vi "Window-Restart window.vi"(8 "error in (no error)":errorcluster) -> (0 "error out":errorcluster, 1 "Cancelled (Left button pressed)":bool)   [LabVIEW 2017]
doc: "Use this template to create a dialog box with event handling."
uses:
  <vilib>/Utility/miscctls.llb/LVPointTypeDef.ctl
  Global Variables/General Globals.vi
panel:
  in  "Left Button":bool
  in  "Rigth Button":bool
  # "Confirm software restart"
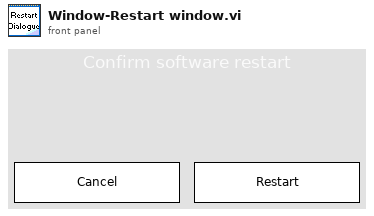
[diagram p1: front panel]
types:
  T1 = typedef "LVPointTypeDef.ctl" = cluster{"Horizontal":i16, "Vertical":i16}
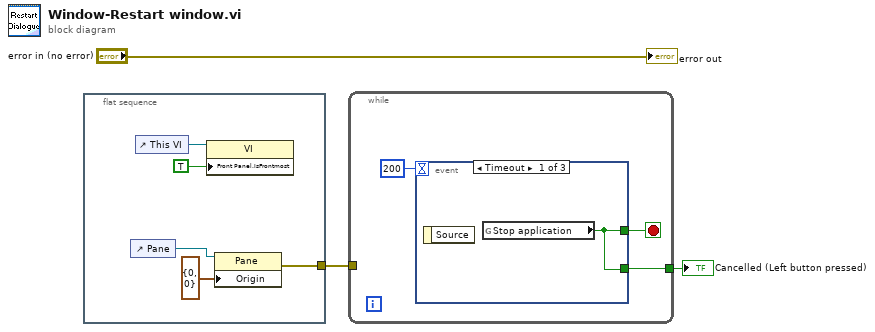
[diagram p0: block diagram]
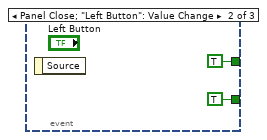
[diagram p2: hidden frame]
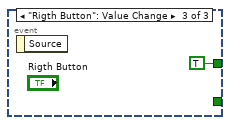
[diagram p3: hidden frame]
diagram:
  n1 = flat-sequence {
    tunnel: [w5] -> w3
    frame #0 {
      n2 = control-ref of="Pane"() -> (w4:refnum<vi>)
      n3 = control-ref of="This VI"() -> (w7:refnum<vi>)
      n4 = property on="Property Node" class="VI"(reference=w7, "Front Panel.IsFrontmost"=TRUE ("Front Panel Window:Is Frontmost")) -> ()  [unwired: 1 in, 2 out]
      n5 = property class="Pane"(reference=w4, "Origin"=T1 {"Horizontal"=0, "Vertical"=0}) -> (error out=w5:errorcluster)  [unwired: 1 in, 1 out]
    }
  }
  n6 = while {
    tunnel: w3 -> [_]
    tunnel: [w9] -> w2
    stop <- w11 stop-if-true
    n7 = event shown="[0] Timeout" {
      selector: _ -> [_ _ _]
      dyn-events: _ -> [_ _ _]
      timeout: 200 -> [_ _ _]
      tunnel: [w12 TRUE ("Stop?") TRUE ("Stop?")] -> w11
      tunnel: [w12 TRUE ("Stop subpanel") _] -> w9
      event Timeout {
        n8 = event-data() -> ()  [unwired: 1 in, 1 out]
        n9 = global read "General Globals.vi" "Stop application"() -> (w12:bool)
      }
      event Panel Close; "Left Button": Value Change {
        n10 = event-data() -> ()  [unwired: 1 in, 1 out]
      }
      event "Rigth Button": Value Change {
        n11 = event-data() -> ()  [unwired: 1 in, 1 out]
      }
    }
  }
  "Cancelled (Left button pressed)" <- w2
  "error out" <- "error in (no error)"
